vi "Lab Panel V5.24.vi"() -> ()   [LabVIEW 2013]
uses:
  <vilib>/Platform/TimedLoop/XDataNode/timing_clust.ctl
  <vilib>/Platform/TimedLoop/XDataNode/nitl_modes.ctl
  <vilib>/Platform/TimedLoop/XDataNode/wakeup.ctl
  Global 1.vi
  Global display 4.vi
  Global display 3.vi
  Global display 1.vi
  Global display 2.vi
  <vilib>/platform/TimedLoop/XDataNode/XDataNode.xnode
  <vilib>/Platform/TimedLoop/XDataNode/XDNodeRunTimeDep.lvlib
panel:
  out "Simulate IND":bool
  out "Amb Tp":dbl format="%#.0f"
  out "Tp Up":dbl
  out "network error":bool
  out "TEMP":bool
  out "AI":bool
  in  "stop all":bool
  in  "ADMIN":bool
  in  "Tab Control 2":T1(tab)
  out "SIG LAB05-2":T2 {"PF" format="%.2f"; "AMPS" format="%.1f"}
  out "SIG LAB05-1":T2 {"PF" format="%.2f"; "AMPS" format="%.1f"}
  out "SIG LAB04-2":T2 {"PF" format="%.2f"; "AMPS" format="%.1f"}
  out "SIG LAB04-1":T2 {"PF" format="%.2f"; "AMPS" format="%.1f"}
  out "SIG LAB03-2":T2 {"PF" format="%.2f"; "AMPS" format="%.1f"}
  out "SIG LAB03-1":T2 {"PF" format="%.2f"; "AMPS" format="%.1f"}
  out "SIG LAB02-2":T2 {"PF" format="%.2f"; "AMPS" format="%.1f"}
  in  "RUN LAB01-1":bool
  in  "O/I  LAB05-1":bool
  in  "O/I  LAB05-2":bool
  in  "O/I  LAB04-1":bool
  in  "O/I  LAB04-2":bool
  in  "O/I  LAB02-1":bool
  in  "O/I  LAB02-2":bool
  in  "O/I  LAB01-2":bool
  in  "O/I  LAB01-1":bool
  in  "O/I  LAB03-1":bool
  in  "RUN LAB05-2":bool
  in  "RUN LAB05-1":bool
  in  "RUN LAB04-2":bool
  in  "RUN LAB04-1":bool
  in  "RUN LAB03-2":bool
  in  "RUN LAB03-1":bool
  in  "RUN LAB02-2":bool
  in  "RUN LAB02-1":bool
  in  "RUN LAB01-2":bool
  in  "SELECT LAB05-2":T3(radio)
  in  "SELECT LAB05-1":T3(radio)
  in  "SELECT LAB04-2":T3(radio)
  in  "SELECT LAB04-1":T3(radio)
  in  "SELECT LAB03-2":T3(radio)
  in  "SELECT LAB03-1":T3(radio)
  in  "SELECT LAB02-2":T3(radio)
  in  "SELECT LAB02-1":T3(radio)
  in  "SELECT LAB01-2":T3(radio)
  in  "SELECT LAB01-1":T3(radio)
  in  "O/I  LAB03-2":bool
  out "SIG LAB01-1":T2 {"PF" format="%.2f"; "AMPS" format="%.1f"}
  out "SIG LAB01-2":T2 {"PF" format="%.2f"; "AMPS" format="%.1f"}
  out "SIG LAB02-1":T2 {"PF" format="%.2f"; "AMPS" format="%.1f"}
  out "DISP LAB05-2":T4 {"MINS" format="%.2g"}
  out "DISP LAB05-1":T4 {"MINS" format="%.2g"}
  out "DISP LAB04-2":T4 {"MINS" format="%.2g"}
  out "DISP LAB04-1":T4 {"MINS" format="%.2g"}
  out "DISP LAB03-2":T4 {"MINS" format="%.2g"}
  out "DISP LAB03-1":T4 {"MINS" format="%.2g"}
  in  "SET LAB05-2":T5={"NAME"="", "DESCRIPTION"="", "CYCLES"=5.0, "T-RISE mins"=0.0, "T-RISE deg C"=0.0} {"CYCLES" min=5.0 step=1.0}
  in  "SET LAB05-1":T5={"NAME"="", "DESCRIPTION"="", "CYCLES"=5.0, "T-RISE mins"=0.0, "T-RISE deg C"=0.0} {"CYCLES" min=5.0 step=1.0}
  in  "SET LAB04-2":T5={"NAME"="", "DESCRIPTION"="", "CYCLES"=5.0, "T-RISE mins"=0.0, "T-RISE deg C"=0.0} {"CYCLES" min=5.0 step=1.0}
  in  "SET LAB04-1":T5={"NAME"="", "DESCRIPTION"="", "CYCLES"=5.0, "T-RISE mins"=0.0, "T-RISE deg C"=0.0} {"CYCLES" min=5.0 step=1.0}
  in  "SET LAB03-2":T5={"NAME"="", "DESCRIPTION"="", "CYCLES"=5.0, "T-RISE mins"=0.0, "T-RISE deg C"=0.0} {"CYCLES" min=5.0 step=1.0}
  in  "SET LAB03-1":T5={"NAME"="", "DESCRIPTION"="", "CYCLES"=5.0, "T-RISE mins"=0.0, "T-RISE deg C"=0.0} {"CYCLES" min=5.0 step=1.0}
  out "DISP LAB02-2":T4 {"MINS" format="%.2g"}
  out "DISP LAB02-1":T4 {"MINS" format="%.2g"}
  in  "SET LAB02-2":T5={"NAME"="", "DESCRIPTION"="", "CYCLES"=5.0, "T-RISE mins"=0.0, "T-RISE deg C"=0.0} {"CYCLES" min=5.0 step=1.0}
  in  "SET LAB02-1":T5={"NAME"="", "DESCRIPTION"="", "CYCLES"=5.0, "T-RISE mins"=0.0, "T-RISE deg C"=0.0} {"CYCLES" min=5.0 step=1.0}
  out "RESULT LAB05-2":bool
  out "RESULT LAB05-1":bool
  out "RESULT LAB04-2":bool
  out "RESULT LAB04-1":bool
  out "RESULT LAB03-2":bool
  out "RESULT LAB03-1":bool
  out "RESULT LAB02-2":bool
  out "RESULT LAB02-1":bool
  out "RESULT LAB01-2":bool
  out "RESULT LAB01-1":bool
  in  "SET LAB01-1":T5={"NAME"="", "DESCRIPTION"="", "CYCLES"=5.0, "T-RISE mins"=0.0, "T-RISE deg C"=0.0} {"CYCLES" min=5.0 step=1.0}
  in  "SET LAB01-2":T5={"NAME"="", "DESCRIPTION"="", "CYCLES"=5.0, "T-RISE mins"=0.0, "T-RISE deg C"=0.0} {"CYCLES" min=5.0 step=1.0}
  out "DISP LAB01-1":T4 {"MINS" format="%.2g"}
  out "DISP LAB01-2":T4 {"MINS" format="%.2f"}
  out "TEMP RISE LAB05-2":cluster{"TL":dbl, "TN":dbl}
  out "TEMP RISE LAB05-1":cluster{"TL":dbl, "TN":dbl}
  out "TEMP RISE LAB04-2":cluster{"TL":dbl, "TN":dbl}
  out "TEMP RISE LAB04-1":cluster{"TL":dbl, "TN":dbl}
  out "TEMP RISE LAB03-2":cluster{"TL":dbl, "TN":dbl}
  out "TEMP RISE LAB03-1":cluster{"TL":dbl, "TN":dbl}
  out "TEMP RISE LAB02-2":cluster{"TL":dbl, "TN":dbl}
  out "TEMP RISE LAB02-1":cluster{"TL":dbl, "TN":dbl}
  out "TEMP RISE LAB01-2":cluster{"TL":dbl, "TN":dbl}
  out "TEMP RISE LAB01-1":cluster{"TL":dbl, "TN":dbl}
  out "JIG LAB05-2":bool
  out "JIG LAB05-1":bool
  out "JIG LAB04-2":bool
  out "JIG LAB04-1":bool
  out "JIG LAB03-2":bool
  out "JIG LAB03-1":bool
  out "JIG LAB02-2":bool
  out "JIG LAB02-1":bool
  out "JIG LAB01-2":bool
  out "JIG LAB01-1":bool
  out "TEMP START LAB01-1":cluster{"TL":dbl, "TN":dbl}
  out "TEMP START LAB02-1":cluster{"TL":dbl, "TN":dbl}
  out "TEMP START LAB03-1":cluster{"TL":dbl, "TN":dbl}
  out "TEMP START LAB04-1":cluster{"TL":dbl, "TN":dbl}
  out "TEMP START LAB01-2":cluster{"TL":dbl, "TN":dbl}
  out "TEMP START LAB02-2":cluster{"TL":dbl, "TN":dbl}
  out "TEMP START LAB03-2":cluster{"TL":dbl, "TN":dbl}
  out "TEMP START LAB04-2":cluster{"TL":dbl, "TN":dbl}
  out "TEMP START LAB05-2":cluster{"TL":dbl, "TN":dbl}
  out "TEMP START LAB05-1":cluster{"TL":dbl, "TN":dbl}
  out "LOG LAB05-2":string
  out "LOG LAB04-2":string
  out "LOG LAB03-2":string
  out "LOG LAB02-2":string
  out "LOG LAB01-2":string
  out "LOG LAB05-1":string
  out "LOG LAB04-1":string
  out "LOG LAB03-1":string
  out "LOG LAB02-1":string
  out "LOG LAB01-1":string
  in  "Tab charts":T6(tab)
  out "LAB01 VOLTS":dynamicdata(graph)
  out "LAB01 AMPS":dynamicdata(graph)
  out "LAB01 deg C":dynamicdata(graph)
  out "LAB02 VOLTS":dynamicdata(graph)
  out "LAB02 AMPS":dynamicdata(graph)
  out "LAB02 deg C":dynamicdata(graph)
  out "LAB03 VOLTS":dynamicdata(graph)
  out "LAB03 AMPS":dynamicdata(graph)
  out "LAB03 deg C":dynamicdata(graph)
  out "LAB04 VOLTS":dynamicdata(graph)
  out "LAB04 AMPS":dynamicdata(graph)
  out "LAB04 deg C":dynamicdata(graph)
  out "LAB05 VOLTS":dynamicdata(graph)
  out "LAB05 AMPS":dynamicdata(graph)
  out "LAB05 deg C":dynamicdata(graph)
  out "Reset Error":bool
  out "Error Temp":bool
  out "Er USB#2":dbl
  out "Er USB#1":dbl
  out "Er USB#0":dbl
  out "Resets Done":dbl
  out "Error USB #2":bool
  out "Error USB #1":bool
  out "Error USB #0":bool
  in  "MAIL SETTINGS":T7
  out "MAIL REPORT":string
  in  "TO (string):":string
  in  "Send Mail Now":bool
  in  "Auto Mail Send":bool
  in  "Network Directory":path
  in  "JIG ON TIME (S)":dbl=1.0 min=1.0 max=10.0 step=0.5 format="%.1g"
  in  "JIG OFF TIME (S)":dbl=2.0 min=2.0 max=10.0 step=0.5 format="%.1g"
  in  "Reset Measuring":bool
  out "JIG RELAY CYCLES":T8
  out "ON L05-2":cluster{"amps":dbl, "volts":dbl, "pf":dbl}
  out "ON L05-1":cluster{"amps":dbl, "volts":dbl, "pf":dbl}
  out "FAIL LAB05-2":cluster{"LO":dbl, "HI":dbl}
  out "FAIL LAB05-1":cluster{"LO":dbl, "HI":dbl}
  out "FAIL LAB04-2":cluster{"LO":dbl, "HI":dbl}
  out "FAIL LAB04-1":cluster{"LO":dbl, "HI":dbl}
  out "FAIL LAB03-2":cluster{"LO":dbl, "HI":dbl}
  out "FAIL LAB03-1":cluster{"LO":dbl, "HI":dbl}
  out "FAIL LAB02-2":cluster{"LO":dbl, "HI":dbl}
  out "FAIL LAB02-1":cluster{"LO":dbl, "HI":dbl}
  out "FAIL LAB01-2":cluster{"LO":dbl, "HI":dbl}
  out "FAIL LAB01-1":cluster{"LO":dbl, "HI":dbl}
  out "ON L01-1":cluster{"amps":dbl, "volts":dbl, "pf":dbl}
  out "ON L01-2":cluster{"amps":dbl, "volts":dbl, "pf":dbl}
  out "ON L02-1":cluster{"amps":dbl, "volts":dbl, "pf":dbl}
  out "ON L02-2":cluster{"amps":dbl, "volts":dbl, "pf":dbl}
  out "ON L03-1":cluster{"amps":dbl, "volts":dbl, "pf":dbl}
  out "ON L03-2":cluster{"amps":dbl, "volts":dbl, "pf":dbl}
  out "ON L04-1":cluster{"amps":dbl, "volts":dbl, "pf":dbl}
  out "ON L04-2":cluster{"amps":dbl, "volts":dbl, "pf":dbl}
  out "TEMP LA05":T9
  out "TEMP LA04":T9
  out "TEMP LA03":T9
  out "TEMP LA02":T9
  out "TEMP LA01":T9
  out "Ref deg C":dbl format="%#.0f"
  out "Temp read loop":dbl
  out "Total USB resets":dbl
  in  "Auto Reset":bool
  in  "Mail Test File To:":string
  in  "Mail Test Fail":bool
  out "graph flag":bool
  in  "Temp Test Cal":dbl
  in  "Amps Fail level":dbl
  in  "Fail Loops":dbl
  out "Save JC":bool
  in  "Simulate":bool
  in  "Temp Value":dbl
  in  "Temp Delay Lps":dbl
  in  "SAMPLES":dbl
  in  "RATE (Hz)":dbl
  in  "JIG TEST":T10
  in  "C drive data root dir":path
  out "run lab05-2":bool
  out "run lab05-1":bool
  out "run lab04-2":bool
  out "run lab04-1":bool
  out "run lab03-2":bool
  out "run lab03-1":bool
  out "run lab02-2":bool
  out "run lab02-1":bool
  out "run lab01-2":bool
  out "run lab01-1":bool
  in  "Tab Control":T11(tab)
  out "LAB01-2 (GRAPH)":dynamicdata(graph)
  out "LAB01-1 (GRAPH)":dynamicdata(graph)
  out "LAB02-2 (GRAPH)":dynamicdata(graph)
  out "LAB02-1 (GRAPH)":dynamicdata(graph)
  out "LAB03-2 (GRAPH)":dynamicdata(graph)
  out "LAB03-1 (GRAPH)":dynamicdata(graph)
  out "LAB04-2 (GRAPH)":dynamicdata(graph)
  out "LAB04-1 (GRAPH)":dynamicdata(graph)
  out "LAB05-2 (GRAPH)":dynamicdata(graph)
  out "LAB05-1 (GRAPH)":dynamicdata(graph)
  out "Any Test Running":bool
  out "Read Time":dbl
  in  "Read Temp":bool
  out "LAB05 TEMP":T12
  out "LAB04 TEMP":T12
  out "LAB02 TEMP":T12
  out "LAB01 TEMP":T12
  out "LAB03 TEMP":T12
  out "LAB05-TP":bool
  out "LAB04-TP":bool
  out "LAB03-TP":bool
  out "LAB02-TP":bool
  out "LAB01-TP":bool
  out "Analog error":bool
  out "USB OUT 0":bool[](array[boolean])
  out "USB OUT 1":bool[](array[boolean])
  out "USB OUT 2":bool[](array[boolean])
  in  "Ambient Volts":dbl format="%.2f"
  in  "PF":dbl min=0.0 max=1.0 step=0.1 format="%#.1f"
  in  "VOLTS":dbl
  in  "OFF amps":dbl min=0.0 max=100.0 step=0.1 format="%#.1f"
  in  "ON amps":dbl
  in  "LAB deg C":T13
  out "AI loop time":dbl format="%.6g"
  out "loops":dbl
  in  "loop  delay(mS)":dbl
  out "on loops":dbl
  out "off loops":dbl
  out "jig cycle":dbl
  out "TDMS LAB01-1":refnum<k34>
  out "data file error":errorcluster
  out "TDMS LAB02-1":refnum<k34>
  out "TDMS LAB01-2":refnum<k34>
  out "TDMS LAB02-2":refnum<k34>
  out "TDMS LAB03-1":refnum<k34>
  out "TDMS LAB03-2":refnum<k34>
  out "TDMS LAB04-1":refnum<k34>
  out "TDMS LAB04-2":refnum<k34>
  out "TDMS LAB05-1":refnum<k34>
  out "TDMS LAB05-2":refnum<k34>
  out "mail control":string
  out "File Time Stamp":timestamp
  in  "stop":bool
  in  "Select COM port":refnum<visa-resource-name>="COM6"
  out "COM port":refnum<visa-resource-name>="COM6"
  out "deg C (volts)":dbl
  out "TEMP REF cal":dbl
  out "CAL LAB01":T14 {"2 (TN) cal" min=0.0 step=0.01 format="%.2f"; "2 (TL) cal" min=0.0 step=0.01 format="%.2f"; "2 (PF) cal" min=0.0 step=0.01 format="%.2f"; "2 (V) cal" min=0.0 step=0.01 format="%.2f"; "2 (A) cal" min=0.0 step=0.01 format="%.2f"; "1 (TN) cal" min=0.0 step=0.01 format="%.2f"; "1 (TL) cal" min=0.0 step=0.01 format="%.2f"; "1 (PF) cal" min=0.0 step=0.01 format="%.2f"; "1 (V) cal" min=0.0 step=0.01 format="%.2f"; "1  (A) cal" min=0.0 step=0.01 format="%.2f"}
  out "CAL LAB03":T14 {"2 (TN) cal" min=0.0 step=0.01 format="%.2f"; "2 (TL) cal" min=0.0 step=0.01 format="%.2f"; "2 (PF) cal" min=0.0 step=0.01 format="%.2f"; "2 (V) cal" min=0.0 step=0.01 format="%.2f"; "2 (A) cal" min=0.0 step=0.01 format="%.2f"; "1 (TN) cal" min=0.0 step=0.01 format="%.2f"; "1 (TL) cal" min=0.0 step=0.01 format="%.2f"; "1 (PF) cal" min=0.0 step=0.01 format="%.2f"; "1 (V) cal" min=0.0 step=0.01 format="%.2f"; "1  (A) cal" min=0.0 step=0.01 format="%.2f"}
  out "CAL LAB02":T15 {"2 (TN) cal" min=0.0 step=0.01 format="%.2f"; "2 (TL) cal" min=0.0 step=0.01 format="%.2f"; "2 (PF) cal" min=0.0 step=0.01 format="%.2f"; "2 (V) cal" min=0.0 step=0.01 format="%.2f"; "2 (A) cal" min=0.0 step=0.01 format="%.2f"; "1 (TN) cal" min=0.0 step=0.01 format="%.2f"; "1 (TL) cal" min=0.0 step=0.01 format="%.2f"; "1 (PF) cal" min=0.0 step=0.01 format="%.2f"; "1 (V) cal" min=0.0 step=0.01 format="%.2f"; "1 (A) cal" min=0.0 step=0.01 format="%.2f"}
  out "CAL LAB05":T14 {"2 (TN) cal" min=0.0 step=0.01 format="%.2f"; "2 (TL) cal" min=0.0 step=0.01 format="%.2f"; "2 (PF) cal" min=0.0 step=0.01 format="%.2f"; "2 (V) cal" min=0.0 step=0.01 format="%.2f"; "2 (A) cal" min=0.0 step=0.01 format="%.2f"; "1 (TN) cal" min=0.0 step=0.01 format="%.2f"; "1 (TL) cal" min=0.0 step=0.01 format="%.2f"; "1 (PF) cal" min=0.0 step=0.01 format="%.2f"; "1 (V) cal" min=0.0 step=0.01 format="%.2f"; "1  (A) cal" min=0.0 step=0.01 format="%.2f"}
  out "CAL LAB04":T14 {"2 (TN) cal" min=0.0 step=0.01 format="%.2f"; "2 (TL) cal" min=0.0 step=0.01 format="%.2f"; "2 (PF) cal" min=0.0 step=0.01 format="%.2f"; "2 (V) cal" min=0.0 step=0.01 format="%.2f"; "2 (A) cal" min=0.0 step=0.01 format="%.2f"; "1 (TN) cal" min=0.0 step=0.01 format="%.2f"; "1 (TL) cal" min=0.0 step=0.01 format="%.2f"; "1 (PF) cal" min=0.0 step=0.01 format="%.2f"; "1 (V) cal" min=0.0 step=0.01 format="%.2f"; "1  (A) cal" min=0.0 step=0.01 format="%.2f"}
  out "cal file error out":errorcluster
  in  "SET (cal)":bool
  # "LAB01"
  # "LAB02"
  # "LAB03"
  # "LAB04"
  # "LAB05"
  # "LAB01"
  # "LAB02"
  # "LAB03"
  # "LAB04"
  # "LAB05"
  # "PANEL ID / DATE / TIME / NAME / DESCRIPTION / CYCLES / TEST TIME / STATUS"
  # "PANEL ID / DATE / TIME / NAME / DESCRIPTION / CYCLES / TEST TIME / STATUS"
  # "(Enter recipients address seperated by comma)"
  # "JIG SET"
  # "Temperature circuits \ndetected at start up."
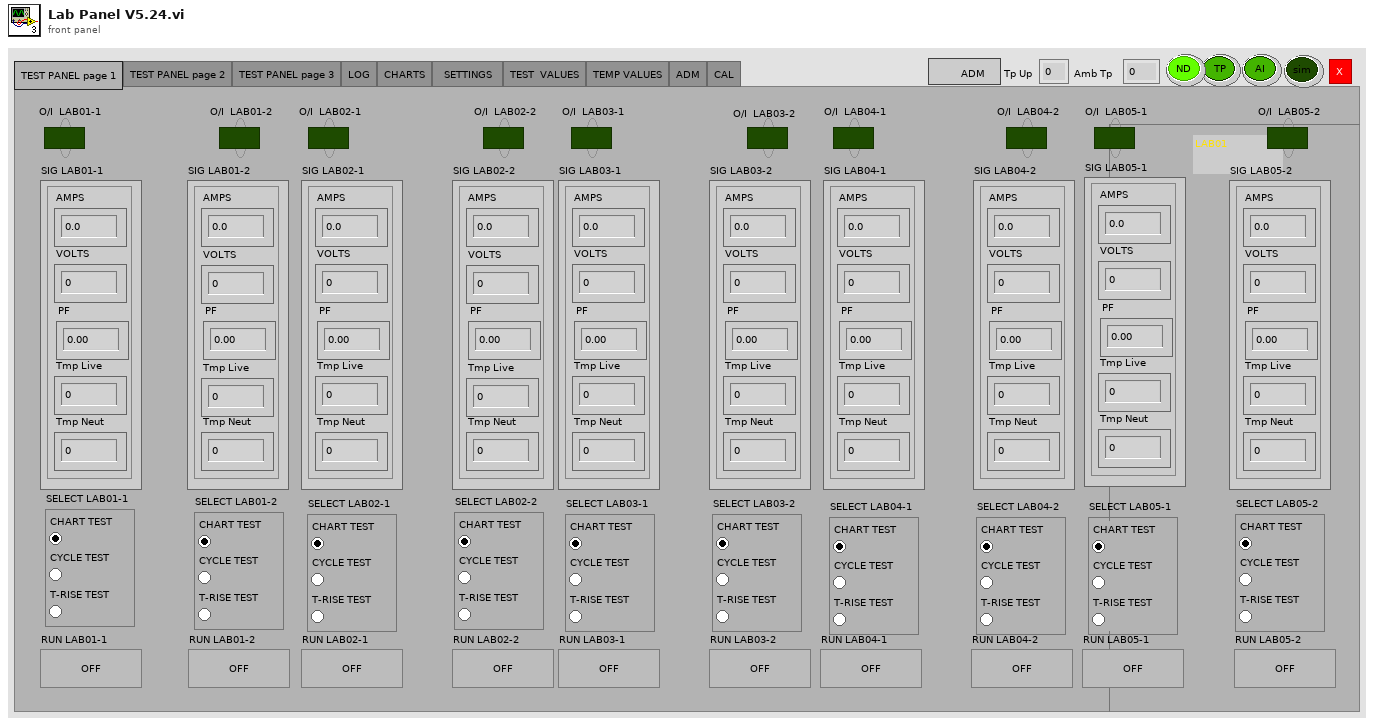
[diagram p1: front panel]
types:
  T1 = enum32{"TEST PANEL page 1", "TEST PANEL page 2", "TEST PANEL page 3", "LOG", "CHARTS", "SETTINGS   ", "TEST  VALUES", "TEMP VALUES", "ADM", "CAL"}
  T2 = cluster{"AMPS":dbl, "VOLTS":dbl, "PF":dbl, "Tmp Live":dbl, "Tmp Neut":dbl}
  T3 = enum32{"CHART TEST", "CYCLE TEST", "T-RISE TEST"}
  T4 = cluster{"CYCLE":dbl, "MINS":dbl, "STATUS":string}
  T5 = cluster{"NAME":string, "DESCRIPTION":string, "CYCLES":dbl, "T-RISE mins":dbl, "T-RISE deg C":dbl}
  T6 = enum32{"LAB01", "LAB02", "LAB03", "LAB04", "LAB05"}
  T7 = cluster{"OUT SERVER ADDRESS":string, "FROM ACCOUNT":string, "USER NAME":string, "PASSWORD":string, "TEST MAIL":bool, "TEST MAIL STATUS":string, "mail error":errorcluster}
  T8 = cluster{"LAB01-1":dbl, "LAB01-2":dbl, "LAB02-1":dbl, "LAB02-2":dbl, "LAB03-1":dbl, "LAB03-2":dbl, "LAB04-1":dbl, "LAB04-2":dbl, "LAB05-1":dbl, "LAB05-2":dbl}
  T9 = cluster{"TL-1":dbl, "TN-1":dbl, "TL-2":dbl, "TN-2":dbl, "TL -1COUNT":dbl, "TN-1 COUNT":dbl, "TL-2 COUNT":dbl, "TN-2 COUNT":dbl}
  T10 = cluster{" LAB01-1":bool, " LAB01-2":bool, "LAB02-1":bool, " LAB02-2":bool, "LAB03-1":bool, "LAB03-2":bool, "LAB04-1":bool, "LAB04-2":bool, "LAB05-1":bool, "LAB05-2":bool}
  T11 = enum32{"LAB01", "LAB02", "LAB03", "LAB04", "LAB05", "TEMPERATURE", "GENERAL INFO", "Simulate"}
  T12 = cluster{"T1 Live":dbl, "T1 Neut":dbl, "T2 Live":dbl, "T2 Neut":dbl, "ID":dbl, "ER":dbl}
  T13 = cluster{"1 TL":dbl, "1 TN":dbl, "2 TL":dbl, "2 TN":dbl, "ID":dbl, "ER":dbl}
  T14 = cluster{"1  (A) cal":dbl, "1 (V) cal":dbl, "1 (PF) cal":dbl, "1 (TL) cal":dbl, "1 (TN) cal":dbl, "2 (A) cal":dbl, "2 (V) cal":dbl, "2 (PF) cal":dbl, "2 (TL) cal":dbl, "2 (TN) cal":dbl}
  T15 = cluster{"1 (A) cal":dbl, "1 (V) cal":dbl, "1 (PF) cal":dbl, "1 (TL) cal":dbl, "1 (TN) cal":dbl, "2 (A) cal":dbl, "2 (V) cal":dbl, "2 (PF) cal":dbl, "2 (TL) cal":dbl, "2 (TN) cal":dbl}
  T16 = enum8{"Enabled", "Disabled", "Disabled and Grayed Out"}
  T17 = enum16{"open", "replace", "create", "open or create", "replace or create", "replace or create with confirmation"}
  T18 = typedef "XDNodeRunTimeDep.lvlib/timing_clust.ctl" = cluster{"Expected End [f-1]":u64, "Actual End [f-1]":u64, "Finished Late? [f-1]":bool, "Expected End [i-1]":u64, "Actual End [i-1]":u64, "Finished Late? [i-1]":bool, "Expected Start [i]":u64, "Actual Start [i]":u64, "Expected Start [f]":u64, "Actual Start [f]":u64, "Source Name":string, "Structure Name":string, "Period":i64, "Deadline":i64, "Offset":i64, "Start":i64, "Priority":i32, "Timeout":i32, "Mode":T19, "Wakeup Reason":T20, "Error":errorcluster, "Source Type":string, "Secondary Source Type":string, "Global End Time":u64, "Global Start Time":u64, "Frame Duration":u64, "Iteration Duration":u64, "Assigned CPU":i32, "I/O Scan Engine Mode":u32}
  T19 = typedef "XDNodeRunTimeDep.lvlib/nitl_modes.ctl" = enum32{"No Change", "Process missed periods, maintain original phase", "Discard missed periods, maintain original phase", "Process missed periods, ignore original phase", "Discard missed periods, ignore original phase"}
  T20 = typedef "XDNodeRunTimeDep.lvlib/wakeup.ctl" = enum32{"Normal", "Aborted", "Asynchronous wakeup", "Timing source error", "Timed loop error", "Timeout"}
  T21 = enum16{"open", "open or create", "create or replace", "create", "open (read-only)"}
  T22 = cluster{"SET LAB01-1":cluster{"NAME":string, "DESCRIPTION":string, "CYCLES":dbl, "T-RISE mins":dbl, "T-RISE deg C":dbl}, "SET LAB01-2":cluster{"NAME":string, "DESCRIPTION":string, "CYCLES":dbl, "T-RISE mins":dbl, "T-RISE deg C":dbl}, "SET LAB02-1":cluster{"NAME":string, "DESCRIPTION":string, "CYCLES":dbl, "T-RISE mins":dbl, "T-RISE deg C":dbl}, "SET LAB02-2":cluster{"NAME":string, "DESCRIPTION":string, "CYCLES":dbl, "T-RISE mins":dbl, "T-RISE deg C":dbl}, "SET LAB03-1":cluster{"NAME":string, "DESCRIPTION":string, "CYCLES":dbl, "T-RISE mins":dbl, "T-RISE deg C":dbl}, "SET LAB03-2":cluster{"NAME":string, "DESCRIPTION":string, "CYCLES":dbl, "T-RISE mins":dbl, "T-RISE deg C":dbl}, "SET LAB04-1":cluster{"NAME":string, "DESCRIPTION":string, "CYCLES":dbl, "T-RISE mins":dbl, "T-RISE deg C":dbl}, "SET LAB04-2":cluster{"NAME":string, "DESCRIPTION":string, "CYCLES":dbl, "T-RISE mins":dbl, "T-RISE deg C":dbl}, "SET LAB05-1":cluster{"NAME":string, "DESCRIPTION":string, "CYCLES":dbl, "T-RISE mins":dbl, "T-RISE deg C":dbl}, "SET LAB05-2":cluster{"NAME":string, "DESCRIPTION":string, "CYCLES":dbl, "T-RISE mins":dbl, "T-RISE deg C":dbl}, "Network Directory":path, "C drive data root dir":path, "RATE (Hz)":dbl, "SAMPLES":dbl, "Select COM port":refnum<visa-resource-name>, "Temp Delay Lps":dbl, "Temp Value":dbl, "Fail Loops":dbl, "Temp Test Cal":dbl, "Amps Fail level":dbl, "Mail Test File To:":string, "Mail Test Fail":bool}
  T23 = cluster{"MAIL SETTINGS":cluster{"OUT SERVER ADDRESS":string, "FROM ACCOUNT":string, "USER NAME":string, "PASSWORD":string, "TEST MAIL":bool, "TEST MAIL STATUS":string, "mail error":errorcluster}, "Auto Mail Send":bool, string}
  T24 = cluster{"id1":bool, "id2":bool, "id3":bool, "id4":bool, "id5":bool}
  T25 = cluster{"T1":dbl, "T2":dbl, "T3":dbl, "T4":dbl, "ID":dbl, "ER":dbl}
  T26 = cluster{"STATUS":string, "OUT SERVER ADDRESS":string, "FROM ACCOUNT":string, "Mail Test File To:":string, "Mail Test Fail":bool}
  T27 = cluster{"LAB01-1 (A)":dbl, "LAB01-1 (V)":dbl, "LAB01-1 (PF)":dbl, "LAB01-2 (A)":dbl, "LAB01-2 (V)":dbl, "LAB01-2 (PF)":dbl}
  T28 = cluster{"LAB02-1 (A)":dbl, "LAB02-1 (V)":dbl, "LAB02-1 (PF)":dbl, "LAB02-2 (A)":dbl, "LAB02-2 (V)":dbl, "LAB02-2 (PF)":dbl}
  T29 = cluster{"LAB03-1 (A)":dbl, "LAB03-1 (V)":dbl, "LAB03-1 (PF)":dbl, "LAB03-2 (A)":dbl, "LAB03-2 (V)":dbl, "LAB03-2 (PF)":dbl}
  T30 = cluster{"LAB04-1 (A)":dbl, "LAB04-1 (V)":dbl, "LAB04-1 (PF)":dbl, "LAB04-2 (A)":dbl, "LAB04-2 (V)":dbl, "LAB04-2 (PF)":dbl}
  T31 = cluster{"LAB05-1 (A)":dbl, "LAB05-1 (V)":dbl, "LAB05-1 (PF)":dbl, "LAB05-2 (A)":dbl, "LAB05-2 (V)":dbl, "LAB05-2 (PF)":dbl}
  T32 = cluster{"OFF amps":dbl, "VOLTS":dbl, "PF":dbl, "OFF amps":dbl, "VOLTS":dbl, "PF":dbl}
  T33 = cluster{"FAIL LAB01-1":cluster{"LO":dbl, "HI":dbl}, "SIG LAB01-1":cluster{"AMPS":dbl, "VOLTS":dbl, "PF":dbl, "Tmp Live":dbl, "Tmp Neut":dbl}, "TEMP START LAB01-1":cluster{"TL":dbl, "TN":dbl}, "DISP LAB01-1":cluster{"CYCLE":dbl, "MINS":dbl, "STATUS":string}, "SET LAB01-1":cluster{"NAME":string, "DESCRIPTION":string, "CYCLES":dbl, "T-RISE mins":dbl, "T-RISE deg C":dbl}, "TDMS LAB01-1":refnum<k34>}
  T34 = cluster{"FAIL LAB01-2":cluster{"LO":dbl, "HI":dbl}, "SIG LAB01-2":cluster{"AMPS":dbl, "VOLTS":dbl, "PF":dbl, "Tmp Live":dbl, "Tmp Neut":dbl}, "TEMP START LAB01-2":cluster{"TL":dbl, "TN":dbl}, "DISP LAB01-2":cluster{"CYCLE":dbl, "MINS":dbl, "STATUS":string}, "SET LAB01-2":cluster{"NAME":string, "DESCRIPTION":string, "CYCLES":dbl, "T-RISE mins":dbl, "T-RISE deg C":dbl}, "TDMS LAB01-2":refnum<k34>}
  T35 = cluster{"FAIL LAB02-1":cluster{"LO":dbl, "HI":dbl}, "SIG LAB02-1":cluster{"AMPS":dbl, "VOLTS":dbl, "PF":dbl, "Tmp Live":dbl, "Tmp Neut":dbl}, "TEMP START LAB02-1":cluster{"TL":dbl, "TN":dbl}, "DISP LAB02-1":cluster{"CYCLE":dbl, "MINS":dbl, "STATUS":string}, "SET LAB02-1":cluster{"NAME":string, "DESCRIPTION":string, "CYCLES":dbl, "T-RISE mins":dbl, "T-RISE deg C":dbl}, "TDMS LAB02-1":refnum<k34>}
  T36 = cluster{"FAIL LAB02-2":cluster{"LO":dbl, "HI":dbl}, "SIG LAB02-2":cluster{"AMPS":dbl, "VOLTS":dbl, "PF":dbl, "Tmp Live":dbl, "Tmp Neut":dbl}, "TEMP START LAB02-2":cluster{"TL":dbl, "TN":dbl}, "DISP LAB02-2":cluster{"CYCLE":dbl, "MINS":dbl, "STATUS":string}, "SET LAB02-2":cluster{"NAME":string, "DESCRIPTION":string, "CYCLES":dbl, "T-RISE mins":dbl, "T-RISE deg C":dbl}, "TDMS LAB02-2":refnum<k34>}
  T37 = cluster{"FAIL LAB03-1":cluster{"LO":dbl, "HI":dbl}, "SIG LAB03-1":cluster{"AMPS":dbl, "VOLTS":dbl, "PF":dbl, "Tmp Live":dbl, "Tmp Neut":dbl}, "TEMP START LAB03-1":cluster{"TL":dbl, "TN":dbl}, "DISP LAB03-1":cluster{"CYCLE":dbl, "MINS":dbl, "STATUS":string}, "SET LAB03-1":cluster{"NAME":string, "DESCRIPTION":string, "CYCLES":dbl, "T-RISE mins":dbl, "T-RISE deg C":dbl}, "TDMS LAB03-1":refnum<k34>}
  T38 = cluster{"FAIL LAB03-2":cluster{"LO":dbl, "HI":dbl}, "SIG LAB03-2":cluster{"AMPS":dbl, "VOLTS":dbl, "PF":dbl, "Tmp Live":dbl, "Tmp Neut":dbl}, "TEMP START LAB03-2":cluster{"TL":dbl, "TN":dbl}, "DISP LAB03-2":cluster{"CYCLE":dbl, "MINS":dbl, "STATUS":string}, "SET LAB03-2":cluster{"NAME":string, "DESCRIPTION":string, "CYCLES":dbl, "T-RISE mins":dbl, "T-RISE deg C":dbl}, "TDMS LAB03-2":refnum<k34>}
  T39 = cluster{"FAIL LAB04-1":cluster{"LO":dbl, "HI":dbl}, "SIG LAB04-1":cluster{"AMPS":dbl, "VOLTS":dbl, "PF":dbl, "Tmp Live":dbl, "Tmp Neut":dbl}, "TEMP START LAB04-1":cluster{"TL":dbl, "TN":dbl}, "DISP LAB04-1":cluster{"CYCLE":dbl, "MINS":dbl, "STATUS":string}, "SET LAB04-1":cluster{"NAME":string, "DESCRIPTION":string, "CYCLES":dbl, "T-RISE mins":dbl, "T-RISE deg C":dbl}, "TDMS LAB04-1":refnum<k34>}
  T40 = cluster{"FAIL LAB04-2":cluster{"LO":dbl, "HI":dbl}, "SIG LAB04-2":cluster{"AMPS":dbl, "VOLTS":dbl, "PF":dbl, "Tmp Live":dbl, "Tmp Neut":dbl}, "TEMP START LAB04-2":cluster{"TL":dbl, "TN":dbl}, "DISP LAB04-2":cluster{"CYCLE":dbl, "MINS":dbl, "STATUS":string}, "SET LAB04-2":cluster{"NAME":string, "DESCRIPTION":string, "CYCLES":dbl, "T-RISE mins":dbl, "T-RISE deg C":dbl}, "TDMS LAB04-2":refnum<k34>}
  T41 = cluster{"FAIL LAB05-1":cluster{"LO":dbl, "HI":dbl}, "SIG LAB05-1":cluster{"AMPS":dbl, "VOLTS":dbl, "PF":dbl, "Tmp Live":dbl, "Tmp Neut":dbl}, "TEMP START LAB05-1":cluster{"TL":dbl, "TN":dbl}, "DISP LAB05-1":cluster{"CYCLE":dbl, "MINS":dbl, "STATUS":string}, "SET LAB05-1":cluster{"NAME":string, "DESCRIPTION":string, "CYCLES":dbl, "T-RISE mins":dbl, "T-RISE deg C":dbl}, "TDMS LAB05-1":refnum<k34>}
  T42 = cluster{"FAIL LAB05-2":cluster{"LO":dbl, "HI":dbl}, "SIG LAB05-2":cluster{"AMPS":dbl, "VOLTS":dbl, "PF":dbl, "Tmp Live":dbl, "Tmp Neut":dbl}, "TEMP START LAB05-2":cluster{"TL":dbl, "TN":dbl}, "DISP LAB05-2":cluster{"CYCLE":dbl, "MINS":dbl, "STATUS":string}, "SET LAB05-2":cluster{"NAME":string, "DESCRIPTION":string, "CYCLES":dbl, "T-RISE mins":dbl, "T-RISE deg C":dbl}, "TDMS LAB05-2":refnum<k34>}
  T43 = cluster{"MAIL SETTINGS":cluster{"OUT SERVER ADDRESS":string, "FROM ACCOUNT":string, "USER NAME":string, "PASSWORD":string, "TEST MAIL":bool, "TEST MAIL STATUS":string, "mail error":errorcluster}, "Auto Mail Send":bool, "TO (string):":string}
  T44 = cluster{"TP1-L":dbl, "TP1-N":dbl, "TP2-L":dbl, "TP2-N":dbl, "TP1-L COUNT":dbl, "TP1-N COUNT":dbl, "TP2-L COUNT":dbl, "TP2-N COUNT":dbl}
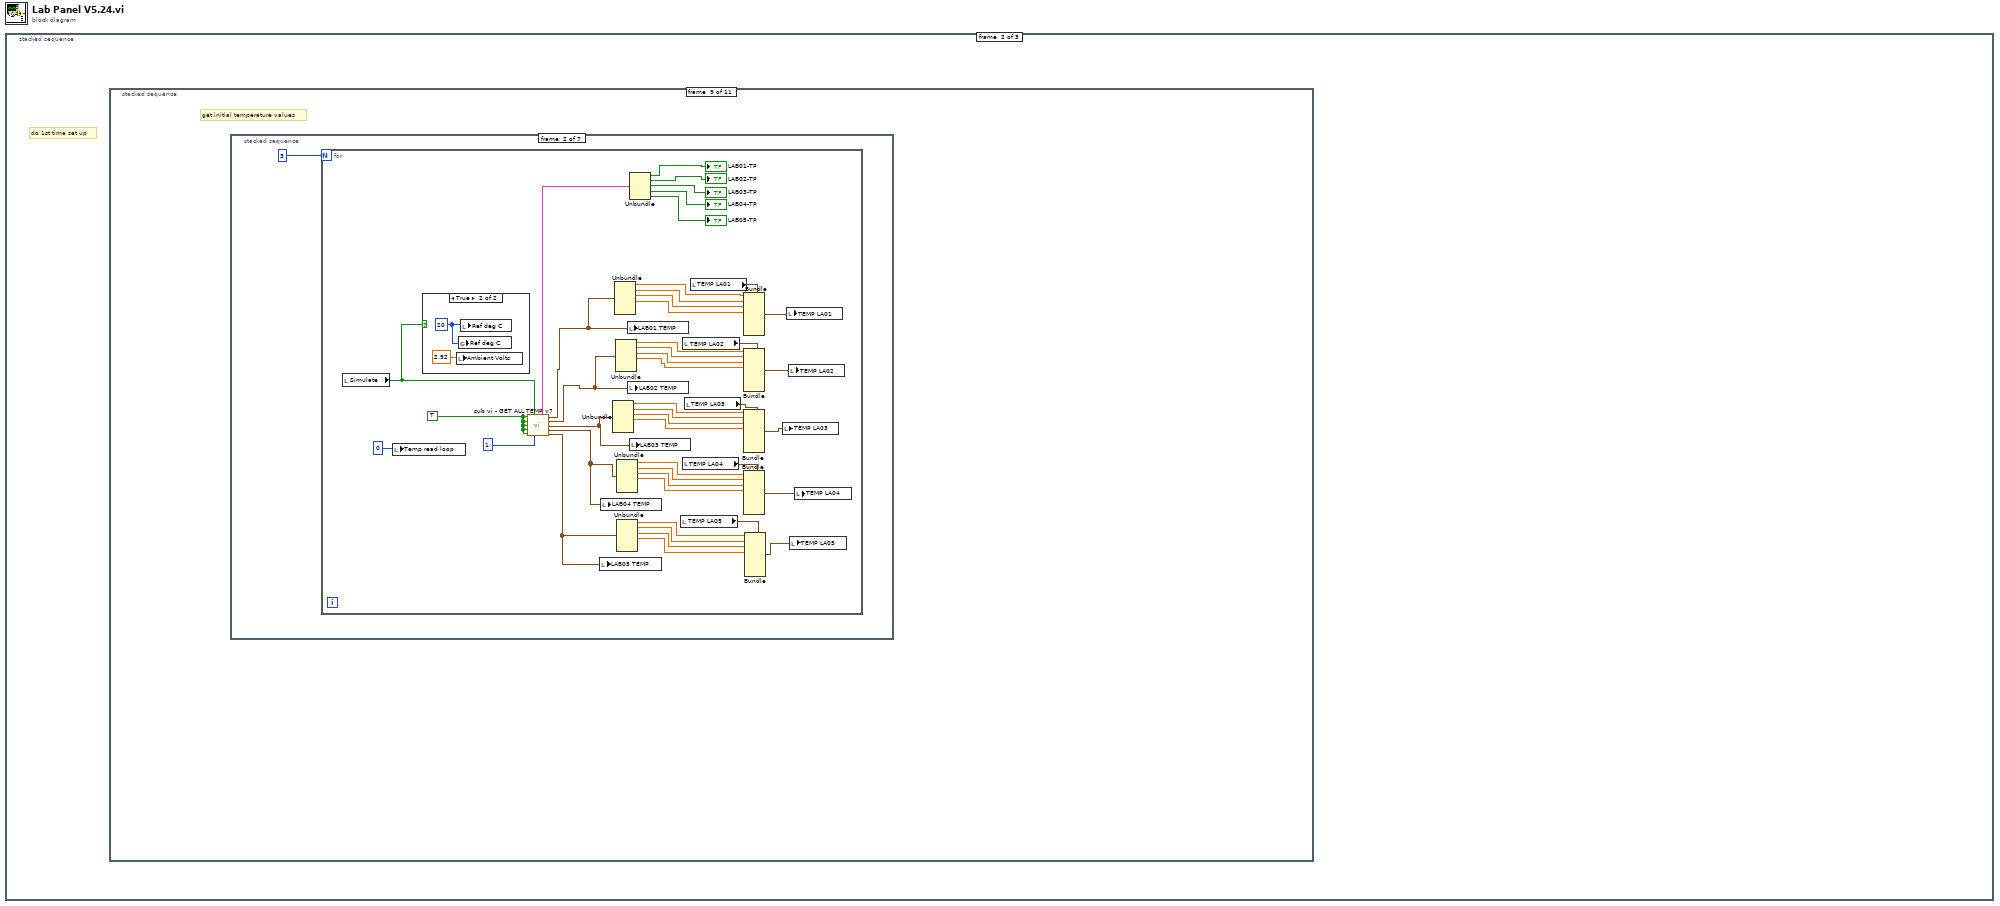
[diagram p0: block diagram]
diagram:
  n1 = stacked-sequence {
    frame #0 {
      n2 = local write "loop  delay(mS)"(500) -> ()
      n3 = local write "Save JC"(FALSE) -> ()
      "jig cycle" <- 0
    }
    frame #1 {
      # "do 1st time set up"
      n4 = stacked-sequence {
        frame #0 {
          # "disable front panel while 1st time set up is being done"
          n5 = disable-structure shown="Enabled" {
            frame Enabled {
              n6 = property on="Tab Control 2" class="TabCtl (strict)"() -> ("Pages"=w10:refnum<vi>[])  [unwired: 2 in, 2 out]
              n7 = Index Array(array=w10, index=8) -> (element=w8:refnum<vi>)
              n8 = property class="Page"(reference=w8, "PageVis"=FALSE) -> ()  [unwired: 1 in, 2 out]
            }
            frame Disabled {
            }
          }
          n9 = property on="Tab Control 2" class="TabCtl (strict)"("Value"=0) -> ()  [unwired: 2 in, 2 out]
          n10 = local write "ADMIN"(FALSE) -> ()
          n11 = property on="Tab Control 2" class="TabCtl (strict)"("DisabledEnum"=T16."Disabled and Grayed Out" ("Disabled")) -> ()  [unwired: 2 in, 2 out]
        }
        frame #1 {
          # "get calibration values"
          n12 = call "sub vi - get calibration values v1.vi"() -> ("TEMP REF CAL"=w11:dbl, "LAB01 (CAL)"=→"CAL LAB01":T14, "LAB02 (CAL)"=→"CAL LAB02":T15, "LAB03 (CAL)"=→"CAL LAB03":T14, "LAB04 (CAL)"=→"CAL LAB04":T14, "calibration file error out"=→"cal file error out":errorcluster, "LAB05 (CAL)"=→"CAL LAB05":T14)  [unwired: 9 in]
          n13 = local write "TEMP REF cal"(w11) -> ()
        }
        frame #2 {
          # "get last saved test settings from file"
          n14 = local read "Network Directory"() -> (w40:path)
          n15 = local read "C drive data root dir"() -> (w38:path)
          n16 = local read "SET LAB05-2"() -> (w70:T5)
          n17 = local read "SET LAB05-1"() -> (w71:T5)
          n18 = local read "SAMPLES"() -> (w36:dbl)
          n19 = local read "SET LAB04-2"() -> (w72:T5)
          n20 = local read "RATE (Hz)"() -> (w37:dbl)
          n21 = local read "SET LAB03-2"() -> (w69:T5)
          n22 = local read "SET LAB04-1"() -> (w73:T5)
          n23 = local read "SET LAB03-1"() -> (w68:T5)
          n24 = local read "SET LAB02-2"() -> (w67:T5)
          n25 = local read "SET LAB02-1"() -> (w66:T5)
          n26 = local read "SET LAB01-2"() -> (w65:T5)
          n27 = local read "SET LAB01-1"() -> (w64:T5)
          n28 = local read "Select COM port"() -> (w33:refnum<visa-resource-name>)
          n29 = local read "Temp Delay Lps"() -> (w32:dbl)
          n30 = local read "Mail Test File To:"() -> (w22:string)
          n31 = local read "Temp Value"() -> (w31:dbl)
          n32 = local read "Temp Test Cal"() -> (w26:dbl)
          n33 = local read "Amps Fail level"() -> (w25:dbl)
          n34 = local read "Fail Loops"() -> (w28:dbl)
          n35 = local read "Mail Test Fail"() -> (w20:bool)
          n36 = Bundle("SET LAB01-1"=w64, "SET LAB01-2"=w65, "SET LAB02-1"=w66, "SET LAB02-2"=w67, "SET LAB03-1"=w68, "SET LAB03-2"=w69, "SET LAB04-1"=w73, "SET LAB04-2"=w72, "SET LAB05-1"=w71, "SET LAB05-2"=w70, "Network Directory"=w40, "C drive data root dir"=w38, "RATE (Hz)"=w37, "SAMPLES"=w36, "Select COM port"=w33, "Temp Delay Lps"=w32, "Temp Value"=w31, "Fail Loops"=w28, "Temp Test Cal"=w26, "Amps Fail level"=w25, "Mail Test File To:"=w22, "Mail Test Fail"=w20) -> (w57:T22)  [unwired: 1 in]
          n37 = String To Path(string="c:\\crabtree\\Set Up\\") -> (path=w61:path)
          n38 = Build Path(base path=w61, name or relative path="settings.bin") -> (appended path=w59:path)
          n39 = Create Folder(path (use dialog)=w61) -> (error out=w63:errorcluster)  [unwired: 2 in, 2 out]
          n40 = call <vilib>:"Clear Errors.vi"("error in (no error)"=w63) -> ()  [unwired: 6 in, 1 out]
          n41 = Open/Create/Replace File(file path (use dialog)=w59) -> (refnum out=w56:refnum<file>, error out=w58:errorcluster)  [unwired: 5 in, 1 out]
          n42 = Read from Binary File(5:w57, 8:w58, 11:w56) -> (0:w53:errorcluster, 2:w55:T22, 3:w54:refnum<file>)  [unwired: 3 in, 1 out]
          n43 = Unbundle(w55) -> ("SET LAB01-1"=w51:T5, "SET LAB01-2"=w50:T5, "SET LAB02-1"=w49:T5, "SET LAB02-2"=w48:T5, "SET LAB03-1"=w47:T5, "SET LAB03-2"=w46:T5, "SET LAB04-1"=w45:T5, "SET LAB04-2"=w44:T5, "SET LAB05-1"=w43:T5, "SET LAB05-2"=w42:T5, "Network Directory"=w41:path, "C drive data root dir"=w39:path, "RATE (Hz)"=w34:dbl, "SAMPLES"=w35:dbl, "Select COM port"=w18:refnum<visa-resource-name>, "Temp Delay Lps"=w30:dbl, "Temp Value"=w29:dbl, "Fail Loops"=w27:dbl, "Temp Test Cal"=w24:dbl, "Amps Fail level"=w23:dbl, "Mail Test File To:"=w21:string, "Mail Test Fail"=w19:bool)
          n44 = Close File(refnum=w54, error in=w53) -> (error out=w52:errorcluster)  [unwired: 1 out]
          n45 = local write "data file error"(w52) -> ()
          n46 = local write "Temp Test Cal"(w24) -> ()
          n47 = local write "Mail Test File To:"(w21) -> ()
          n48 = local write "Amps Fail level"(w23) -> ()
          n49 = local write "Mail Test Fail"(w19) -> ()
          n50 = local write "Fail Loops"(w27) -> ()
          n51 = local write "Temp Delay Lps"(w30) -> ()
          n52 = local write "C drive data root dir"(w39) -> ()
          n53 = local write "Temp Value"(w29) -> ()
          n54 = local write "Network Directory"(w41) -> ()
          n55 = local write "SAMPLES"(w35) -> ()
          n56 = local write "RATE (Hz)"(w34) -> ()
          n57 = local write "SET LAB04-2"(w44) -> ()
          n58 = local write "SET LAB05-1"(w43) -> ()
          n59 = local write "SET LAB04-1"(w45) -> ()
          n60 = local write "SET LAB05-2"(w42) -> ()
          n61 = local write "SET LAB02-1"(w49) -> ()
          n62 = local write "SET LAB02-2"(w48) -> ()
          n63 = local write "SET LAB03-1"(w47) -> ()
          n64 = local write "SET LAB03-2"(w46) -> ()
          n65 = local write "SET LAB01-1"(w51) -> ()
          n66 = local write "SET LAB01-2"(w50) -> ()
          n67 = local write "Select COM port"(w18) -> ()
          n68 = global write "Global 1.vi" "COM port"(w18) -> ()
        }
        frame #3 {
          # "get total resets value from file"
          n69 = String To Path(string="c:\\crabtree\\Set Up\\") -> (path=w84:path)
          n70 = Build Path(base path=w84, name or relative path="USB resets.bin") -> (appended path=w77:path)
          n71 = Create Folder(path (use dialog)=w84) -> (error out=w76:errorcluster)  [unwired: 2 in, 2 out]
          n72 = call <vilib>:"Clear Errors.vi"("error in (no error)"=w76) -> ()  [unwired: 6 in, 1 out]
          n73 = Open/Create/Replace File(file path (use dialog)=w77, operation (0:open)=T17."open or create") -> (refnum out=w82:refnum<file>, error out=w81:errorcluster)  [unwired: 4 in, 1 out]
          n74 = local read "Total USB resets"() -> (w75:dbl)
          n75 = Read from Binary File(5:w75, 8:w81, 11:w82) -> (0:w79:errorcluster, 2:w74:dbl, 3:w80:refnum<file>)  [unwired: 3 in, 1 out]
          n76 = local write "Total USB resets"(w74) -> ()
          n77 = Close File(refnum=w80, error in=w79) -> (error out=w78:errorcluster)  [unwired: 1 out]
          n78 = local write "data file error"(w78) -> ()
        }
        frame #4 {
          # "get last saved jig cycles value from file"
          n79 = String To Path(string="c:\\crabtree\\Jig Cycles\\") -> (path=w96:path)
          n80 = Build Path(base path=w96, name or relative path="jigcycles.bin") -> (appended path=w94:path)
          n81 = Create Folder(path (use dialog)=w96) -> (error out=w98:errorcluster)  [unwired: 2 in, 2 out]
          n82 = call <vilib>:"Clear Errors.vi"("error in (no error)"=w98) -> ()  [unwired: 6 in, 1 out]
          n83 = Open/Create/Replace File(file path (use dialog)=w94) -> (refnum out=w92:refnum<file>, error out=w93:errorcluster)  [unwired: 5 in, 1 out]
          n84 = Read from Binary File(5:T8 {"LAB01-1"=0.0, "LAB01-2"=0.0, "LAB02-1"=0.0, "LAB02-2"=0.0, "LAB03-1"=0.0, "LAB03-2"=0.0, "LAB04-1"=0.0, "LAB04-2"=0.0, "LAB05-1"=0.0, "LAB05-2"=0.0} ("JIG RELAY CYCLES"), 8:w93, 11:w92) -> (0:w90:errorcluster, 2:w87:T8, 3:w91:refnum<file>)  [unwired: 3 in, 1 out]
          n85 = local write "JIG RELAY CYCLES"(w87) -> ()
          n86 = Close File(refnum=w91, error in=w90) -> (error out=w89:errorcluster)  [unwired: 1 out]
          n87 = local write "data file error"(w89) -> ()
        }
        frame #5 {
          # "get mail settings"
          n88 = local read "Auto Mail Send"() -> (w102:bool)
          n89 = local read "MAIL SETTINGS"() -> (w106:T7)
          n90 = String To Path(string="c:\\crabtree\\Set Up\\") -> (path=w114:path)
          n91 = Build Path(base path=w114, name or relative path="mail.bin") -> (appended path=w112:path)
          n92 = Create Folder(path (use dialog)=w114) -> (error out=w116:errorcluster)  [unwired: 2 in, 2 out]
          n93 = Bundle("MAIL SETTINGS"=w106, "Auto Mail Send"=w102, "") -> (w105:T23)  [unwired: 1 in]
          n94 = call <vilib>:"Clear Errors.vi"("error in (no error)"=w116) -> ()  [unwired: 6 in, 1 out]
          n95 = Open/Create/Replace File(file path (use dialog)=w112) -> (refnum out=w110:refnum<file>, error out=w111:errorcluster)  [unwired: 5 in, 1 out]
          n96 = Read from Binary File(5:w105, 8:w111, 11:w110) -> (0:w108:errorcluster, 2:w104:T23, 3:w109:refnum<file>)  [unwired: 3 in, 1 out]
          n97 = Unbundle(w104) -> ("MAIL SETTINGS"=w103:T7, "Auto Mail Send"=w101:bool, w100:string)
          n98 = local write "TO (string):"(w100) -> ()
          n99 = local write "Auto Mail Send"(w101) -> ()
          n100 = local write "MAIL SETTINGS"(w103) -> ()
          n101 = Close File(refnum=w109, error in=w108) -> (error out=w107:errorcluster)  [unwired: 1 out]
          n102 = local write "data file error"(w107) -> ()
        }
        frame #6 {
          # "set display status if blank"
          n103 = local read "DISP LAB03-2"() -> (w146:T4)
          n104 = local read "DISP LAB03-1"() -> (w153:T4)
          n105 = local read "DISP LAB02-2"() -> (w160:T4)
          n106 = local read "DISP LAB01-2"() -> (w173:T4)
          n107 = local read "DISP LAB01-1"() -> (w182:T4)
          n108 = local read "DISP LAB02-1"() -> (w167:T4)
          n109 = Unbundle(w146) -> ("STATUS"=w148:string)  [unwired: 2 out]
          n110 = Unbundle(w153) -> ("STATUS"=w155:string)  [unwired: 2 out]
          n111 = Unbundle(w160) -> ("STATUS"=w162:string)  [unwired: 2 out]
          n112 = Unbundle(w167) -> ("STATUS"=w169:string)  [unwired: 2 out]
          n113 = Unbundle(w173) -> ("STATUS"=w176:string)  [unwired: 2 out]
          n114 = Unbundle(w182) -> ("STATUS"=w183:string)  [unwired: 2 out]
          n115 = Equal?(x="", y=w148) -> (x = y?=w150:bool)
          n116 = Equal?(x="", y=w155) -> (x = y?=w157:bool)
          n117 = Equal?(x="", y=w162) -> (x = y?=w164:bool)
          n118 = Equal?(x="", y=w169) -> (x = y?=w171:bool)
          n119 = Equal?(x="", y=w176) -> (x = y?=w178:bool)
          n120 = Equal?(x="", y=w183) -> (x = y?=w185:bool)
          n121 = Select(t="STOP", s=w150, f=w148) -> (s? t:f=w147:string)
          n122 = Select(t="STOP", s=w157, f=w155) -> (s? t:f=w154:string)
          n123 = Select(t="STOP", s=w164, f=w162) -> (s? t:f=w161:string)
          n124 = Select(t="STOP", s=w171, f=w169) -> (s? t:f=w168:string)
          n125 = Select(t="STOP", s=w178, f=w176) -> (s? t:f=w175:string)
          n126 = Select(t="STOP", s=w185, f=w183) -> (s? t:f=w181:string)
          n127 = Bundle(cluster=w146, "STATUS"=w147) -> (w145:T4)  [unwired: 2 in]
          n128 = Bundle(cluster=w153, "STATUS"=w154) -> (w152:T4)  [unwired: 2 in]
          n129 = Bundle(cluster=w160, "STATUS"=w161) -> (w159:T4)  [unwired: 2 in]
          n130 = Bundle(cluster=w167, "STATUS"=w168) -> (w166:T4)  [unwired: 2 in]
          n131 = Bundle(cluster=w173, "STATUS"=w175) -> (w174:T4)  [unwired: 2 in]
          n132 = Bundle(cluster=w182, "STATUS"=w181) -> (w180:T4)  [unwired: 2 in]
          n133 = local write "DISP LAB01-2"(w174) -> ()
          n134 = local write "DISP LAB01-1"(w180) -> ()
          n135 = local write "DISP LAB02-1"(w166) -> ()
          n136 = local write "DISP LAB03-1"(w152) -> ()
          n137 = local write "DISP LAB02-2"(w159) -> ()
          n138 = local write "DISP LAB03-2"(w145) -> ()
          n139 = local read "DISP LAB05-2"() -> (w118:T4)
          n140 = local read "DISP LAB05-1"() -> (w125:T4)
          n141 = local read "DISP LAB04-2"() -> (w127:T4)
          n142 = local read "DISP LAB04-1"() -> (w129:T4)
          n143 = Unbundle(w118) -> ("STATUS"=w120:string)  [unwired: 2 out]
          n144 = Unbundle(w125) -> ("STATUS"=w131:string)  [unwired: 2 out]
          n145 = Unbundle(w127) -> ("STATUS"=w136:string)  [unwired: 2 out]
          n146 = Unbundle(w129) -> ("STATUS"=w141:string)  [unwired: 2 out]
          n147 = Equal?(x="", y=w120) -> (x = y?=w122:bool)
          n148 = Equal?(x="", y=w131) -> (x = y?=w133:bool)
          n149 = Equal?(x="", y=w136) -> (x = y?=w138:bool)
          n150 = Equal?(x="", y=w141) -> (x = y?=w143:bool)
          n151 = Select(t="STOP", s=w122, f=w120) -> (s? t:f=w119:string)
          n152 = Select(t="STOP", s=w133, f=w131) -> (s? t:f=w130:string)
          n153 = Select(t="STOP", s=w138, f=w136) -> (s? t:f=w135:string)
          n154 = Select(t="STOP", s=w143, f=w141) -> (s? t:f=w140:string)
          n155 = Bundle(cluster=w118, "STATUS"=w119) -> (w117:T4)  [unwired: 2 in]
          n156 = Bundle(cluster=w125, "STATUS"=w130) -> (w124:T4)  [unwired: 2 in]
          n157 = Bundle(cluster=w127, "STATUS"=w135) -> (w126:T4)  [unwired: 2 in]
          n158 = Bundle(cluster=w129, "STATUS"=w140) -> (w128:T4)  [unwired: 2 in]
          n159 = local write "DISP LAB05-2"(w117) -> ()
          n160 = local write "DISP LAB05-1"(w124) -> ()
          n161 = local write "DISP LAB04-1"(w128) -> ()
          n162 = local write "DISP LAB04-2"(w126) -> ()
        }
        frame #7 {
          # "initialise analog input express vi's"
          n163 = for {
            N: 4.0 -> [_]
            w191 = 0
            w189 = FALSE
            n164 = call "sub vi - analog 1st setup v1.vi"() -> ()  [unwired: 9 in, 7 out]
            n165 = local write "Resets Done"(0) -> ()
            n166 = local write "Auto Reset"(TRUE) -> ()
            n167 = local write "Er USB#0"(w191) -> ()
            n168 = local write "Er USB#1"(w191) -> ()
            n169 = local write "Er USB#2"(w191) -> ()
            n170 = local write "Analog error"(w189) -> ()
            n171 = local write "Reset Measuring"(w189) -> ()
            n172 = local write "Error USB #0"(w189) -> ()
            n173 = local write "Reset Error"(w189) -> ()
            n174 = local write "Error USB #1"(w189) -> ()
            n175 = local write "Error USB #2"(w189) -> ()
          }
        }
        frame #8 {
          # "get initial temperature values"
          n176 = stacked-sequence {
            frame #0 {
              w196 = T12 {"T1 Live"=20.0, "T1 Neut"=20.0, "T2 Live"=20.0, "T2 Neut"=20.0, "ID"=6.0, "ER"=10.0} ("LAB01 TEMP")
              n177 = local write "LAB deg C"(w196) -> ()
              n178 = global write "Global display 4.vi" "LAB deg C"(w196) -> ()
              n179 = local write "OFF amps"(1.5) -> ()
              n180 = local write "ON amps"(20.0) -> ()
              n181 = local write "VOLTS"(250.0) -> ()
              n182 = local write "PF"(0.5) -> ()
            }
            frame #1 {
              n183 = for {
                N: 3 -> [_]
                w242 = TRUE
                n184 = local read "Simulate"() -> (w204:bool)
                n185 = local write "Temp read loop"(0) -> ()
                n186 = case shown="True" w204 {
                  frame False {
                  }
                  frame True {
                    w244 = 20
                    n187 = local write "Ambient Volts"(2.92) -> ()
                    n188 = global write "Global display 3.vi" "Ref deg C"(w244) -> ()
                    n189 = local write "Ref deg C"(w244) -> ()
                  }
                }
                n190 = call "sub vi - GET ALL TEMP v7.vi"("LA01-EN"=w242, "simulate"=w204, "LA02-EN"=w242, "LA03-EN"=w242, "LA04-EN"=w242, "LA05-EN"=w242, "Gen Cal Value"=1) -> ("ID"=w203:T24, "LA01 TEMP"=w240:T25, "LA02 TEMP"=w233:T25, "LA03 TEMP"=w226:T25, "LA04 TEMP"=w219:T25, "LA05 TEMP"=w212:T25)  [unwired: 1 in, 2 out]
                n191 = local write "LAB05 TEMP"(w212) -> ()
                n192 = local write "LAB04 TEMP"(w219) -> ()
                n193 = Unbundle(w226) -> ("T1"=w223:dbl, "T2"=w222:dbl, "T3"=w221:dbl, "T4"=w220:dbl)  [unwired: 2 out]
                n194 = Unbundle(w240) -> ("T1"=w238:dbl, "T2"=w237:dbl, "T3"=w236:dbl, "T4"=w235:dbl)  [unwired: 2 out]
                n195 = Unbundle(w233) -> ("T1"=w230:dbl, "T2"=w229:dbl, "T3"=w228:dbl, "T4"=w227:dbl)  [unwired: 2 out]
                n196 = Unbundle(w219) -> ("T1"=w217:dbl, "T2"=w216:dbl, "T3"=w215:dbl, "T4"=w214:dbl)  [unwired: 2 out]
                n197 = Unbundle(w212) -> ("T1"=w210:dbl, "T2"=w209:dbl, "T3"=w208:dbl, "T4"=w207:dbl)  [unwired: 2 out]
                n198 = local write "LAB01 TEMP"(w240) -> ()
                n199 = local write "LAB02 TEMP"(w233) -> ()
                n200 = local write "LAB03 TEMP"(w226) -> ()
